vi "Evaluate Part 1.vi"() -> ()   [LabVIEW 2021]
uses:
  Proto/Heat Map.lvclass
panel:
  out "Min Heat":i32
  in  "Input":string
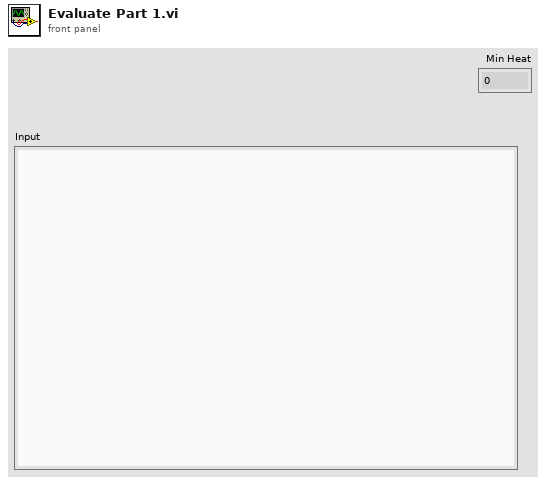
[diagram p1: front panel]
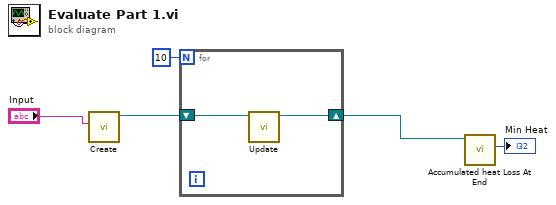
[diagram p0: block diagram]
diagram:
  n1 = call "Create.vi"("Input"="Input") -> ("Proto"=w4:refnum<class "Heat Map.lvclass">)  [unwired: 10 in]
  n2 = for {
    N: 10 -> [_]
    shift-right: [w6] -> w3
    shift-left: w4 -> [w7]
    n3 = call "Update.vi"("Proto in"=w7) -> ("Proto out"=w6:refnum<class "Heat Map.lvclass">)  [unwired: 9 in, 1 out]
  }
  n4 = call "Accumulated heat Loss At End.vi"("Proto in"=w3) -> ("Min Heat"=→"Min Heat":i32)  [unwired: 9 in, 1 out]
